vi "getSequenceStepTimeouts.vi"(7 "error in":errorcluster, 8 "enables":T2, 9 "Slave Address (7-bit)":u8, 10 "I2C Ref In":T3) -> (0 "error out":errorcluster, 2 "timeouts":T1, 3 "I2C Ref Out":T3)   [LabVIEW 2018]
uses:
  <vilib>/myRIO/Instrument Drivers/Onboard IO/I2C/typedefs/I2C Reference.ctl
  <vilib>/myRIO/Common/Instrument Driver Framework/Utilities/typedefs/myRIO Generic Hardware Reference.ctl
  <vilib>/myRIO/Common/Instrument Driver Framework/Utilities/typedefs/Hardware Version Enum.ctl
  <vilib>/myRIO/Common/Instrument Driver Framework/Utilities/typedefs/myRIO v1.0 Reference.ctl
  <vilib>/myRIO/Common/Instrument Driver Framework/Utilities/typedefs/Generic FPGA Reference.ctl
  <vilib>/myRIO/Common/Instrument Driver Framework/myRIO v1.0/I2C/typedefs/I2C Channels Enum.ctl
  <vilib>/myRIO/Instrument Drivers/Onboard IO/I2C/typedefs/I2C Configuration.ctl
  <vilib>/myRIO/Instrument Drivers/Onboard IO/I2C/typedefs/I2C Transfer Rate.ctl
  <vilib>/Utility/error.llb/Error Cluster From Error Code.vi
  <vilib>/myRIO/Common/Instrument Driver Framework/myRIO v1.0/I2C/vis/myRIO v1.0 Write I2C.vi
  <vilib>/myRIO/Common/Instrument Driver Framework/myRIO v1.0/I2C/vis/myRIO v1.0 Read I2C.vi
  <vilib>/myRIO/Instrument Drivers/Onboard IO/I2C/I2C.lvlib
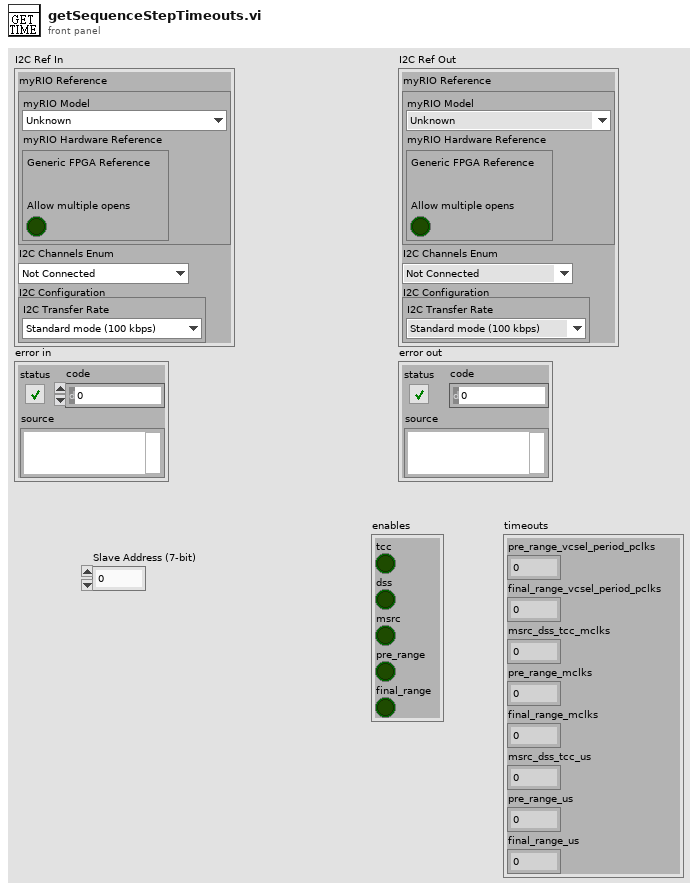
[diagram p1: front panel]
types:
  T1 = cluster{"pre_range_vcsel_period_pclks":u16, "final_range_vcsel_period_pclks":u16, "msrc_dss_tcc_mclks":u16, "pre_range_mclks":u16, "final_range_mclks":u16, "msrc_dss_tcc_us":u32, "pre_range_us":u32, "final_range_us":u32}
  T2 = cluster{"tcc":bool, "dss":bool, "msrc":bool, "pre_range":bool, "final_range":bool}
  T3 = typedef "I2C.lvlib/I2C Reference.ctl" = cluster{"myRIO Reference":T4, "I2C Channels Enum":T8, "I2C Configuration":T9}
  T4 = typedef "myRIO Generic Hardware Reference.ctl" = cluster{"myRIO Model":T5, "myRIO Hardware Reference":T6}
  T5 = typedef "Hardware Version Enum.ctl" = enum16{"Unknown", "myRIO-1900", "myRIO-1950", "roboRIO", "NI ELVIS RIO CM", "ELVIS III"}
  T6 = typedef "myRIO v1.0 Reference.ctl" = cluster{"Generic FPGA Reference":T7, "Allow multiple opens":bool}
  T7 = typedef "Generic FPGA Reference.ctl" = refnum<k20>
  T8 = typedef "I2C Channels Enum.ctl" = enum16{"Not Connected", "A/I2C", "B/I2C", "I2C/I2C"}
  T9 = typedef "I2C.lvlib/I2C Configuration.ctl" = cluster{"I2C Transfer Rate":T10}
  T10 = typedef "I2C.lvlib/I2C Transfer Rate.ctl" = enum16{"Standard mode (100 kbps)", "Fast mode (400 kbps)"}
  T11 = enum8{"VcselPeriodPreRange", "VcselPeriodFinalRange"}
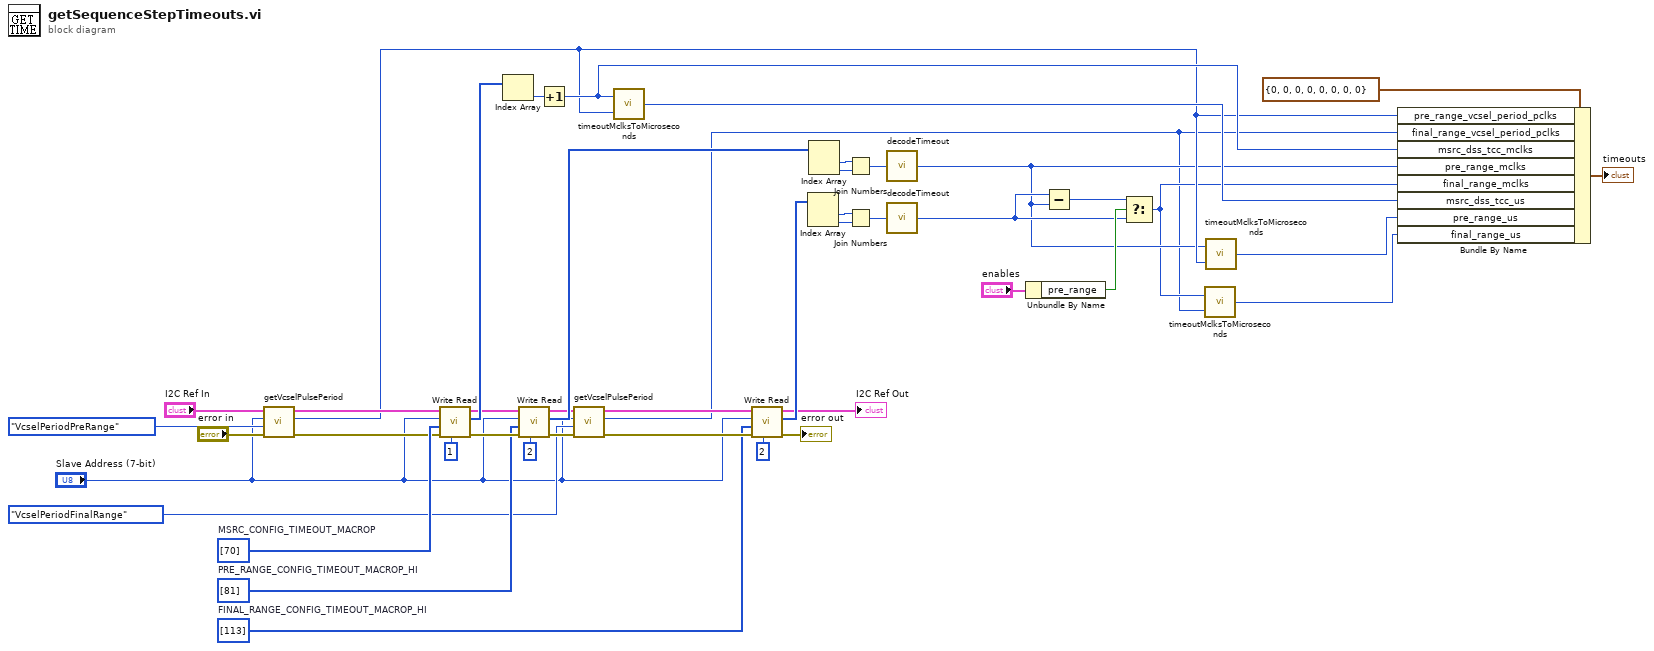
[diagram p0: block diagram]
diagram:
  w17 = u8[] [113]  # FINAL_RANGE_CONFIG_TIMEOUT_MACROP_HI
  w31 = u8[] [81]  # PRE_RANGE_CONFIG_TIMEOUT_MACROP_HI
  w43 = u8[] [70]  # MSRC_CONFIG_TIMEOUT_MACROP
  n1 = call "getVcselPulsePeriod.vi"("error in"="error in", "vcselPeriodType"=T11."VcselPeriodPreRange", "Slave Address (7-bit)"="Slave Address (7-bit)", "I2C Ref In"="I2C Ref In") -> ("error out"=w36:errorcluster, "VcselPulsePeriod"=w25:u8, "I2C Ref Out"=w37:T3)  [unwired: 5 in]
  n2 = call <vilib>:"Write Read.vi"("Byte Count"=u32 1, "error in (no error)"=w36, "Bytes to Write"=w43, "Slave Address (7-bit)"="Slave Address (7-bit)", "I2C Ref In"=w37) -> ("error out"=w33:errorcluster, "Bytes Read"=w44:u8[], "I2C Ref Out"=w34:T3)  [unwired: 3 in]
  n3 = Index Array(array=w44) -> (element=w38:u8)  [unwired: 1 in]
  n4 = call <vilib>:"Write Read.vi"("Byte Count"=u32 2, "error in (no error)"=w33, "Bytes to Write"=w31, "Slave Address (7-bit)"="Slave Address (7-bit)", "I2C Ref In"=w34) -> ("error out"=w22:errorcluster, "Bytes Read"=w30:u8[], "I2C Ref Out"=w23:T3)  [unwired: 3 in]
  n5 = Increment(x=w38) -> (x+1=w27:u8)
  n6 = call "getVcselPulsePeriod.vi"("error in"=w22, "vcselPeriodType"=T11."VcselPeriodFinalRange", "Slave Address (7-bit)"="Slave Address (7-bit)", "I2C Ref In"=w23) -> ("error out"=w19:errorcluster, "VcselPulsePeriod"=w5:u8, "I2C Ref Out"=w20:T3)  [unwired: 5 in]
  n7 = call "timeoutMclksToMicroseconds.vi"("vcsel_period_pclks"=w25, "timeout_period_mclks"=w27) -> ("timeout_period_us"=w35:u32)
  n8 = call <vilib>:"Write Read.vi"("Byte Count"=u32 2, "error in (no error)"=w19, "Bytes to Write"=w17, "Slave Address (7-bit)"="Slave Address (7-bit)", "I2C Ref In"=w20) -> ("error out"=→"error out":errorcluster, "Bytes Read"=w15:u8[], "I2C Ref Out"=→"I2C Ref Out":T3)  [unwired: 3 in]
  n9 = Index Array(array=w15) -> (element #1=w14:u8, element #2=w13:u8)  [unwired: 2 in]
  n10 = Index Array(array=w30) -> (element #1=w28:u8, element #2=w29:u8)  [unwired: 2 in]
  n11 = Join Numbers(hi=w28, lo=w29) -> ((hi.lo)=w26:u16)
  n12 = Join Numbers(hi=w14, lo=w13) -> ((hi.lo)=w12:u16)
  n13 = call "decodeTimeout.vi"("reg_val"=w26) -> ("timeout_mclks"=w8:u16)
  n14 = call "decodeTimeout.vi"("reg_val"=w12) -> ("timeout_mclks"=w9:u16)
  n15 = Unbundle By Name("enables") -> ("pre_range"=w10:bool)
  n16 = Subtract(x=w9, y=w8) -> (x-y=w7:u16)
  n17 = Select(t=w7, s=w10, f=w9) -> (s? t:f=w6:u16)
  n18 = call "timeoutMclksToMicroseconds.vi"("vcsel_period_pclks"=w5, "timeout_period_mclks"=w6) -> ("timeout_period_us"=w4:u32)
  n19 = call "timeoutMclksToMicroseconds.vi"("vcsel_period_pclks"=w25, "timeout_period_mclks"=w8) -> ("timeout_period_us"=w24:u32)
  n20 = Bundle By Name(cluster=T1 {"pre_range_vcsel_period_pclks"=0, "final_range_vcsel_period_pclks"=0, "msrc_dss_tcc_mclks"=0, "pre_range_mclks"=0, "final_range_mclks"=0, "msrc_dss_tcc_us"=0, "pre_range_us"=0, "final_range_us"=0}, "pre_range_vcsel_period_pclks"=w25, "final_range_vcsel_period_pclks"=w5, "msrc_dss_tcc_mclks"=w27, "pre_range_mclks"=w8, "final_range_mclks"=w6, "msrc_dss_tcc_us"=w35, "pre_range_us"=w24, "final_range_us"=w4) -> (→"timeouts":T1)
